vi "Faulhaber_Standalone.vi"() -> ()   [LabVIEW 2011]
panel:
  in  "1:x":i32(slide)=700 scale=-250000.0..250000.0
  in  "Tab Control":enum32{"command", "Script"}(tab)
  in  "commands":cluster{"command":string, "Value":dbl}[](array[cluster])=[{"command"="CONTMOD", "Value"=nan}, {"command"="LR0", "Value"=nan}, {"command"="EN", "Value"=nan}, {"command"="POS", "Value"=nan}, {"command"="OST", "Value"=nan}, {"command"="GAC", "Value"=nan}, {"command"="ac", "Value"=5000.0}, {"command"="GDEC", "Value"=nan}, {"command"="DEC", "Value"=5000.0}, {"command"="GSP", "Value"=nan}, {"command"="SP", "Value"=2500.0}, {"command"="GPOR", "Value"=nan}, {"command"="POR", "Value"=5.0}, {"command"="GI", "Value"=nan}, {"command"="I", "Value"=30.0}, {"command"="GPP", "Value"=nan}, {"command"="PP", "Value"=60.0}, {"command"="GPC", "Value"=nan}, {"command"="LPC", "Value"=500.0}, {"command"="GCC", "Value"=nan}, {"command"="GNL", "Value"=nan}, {"command"="GPL", "Value"=nan}, {"command"="LL", "Value"=12345678.0}, {"command"="TEM", "Value"=nan}, {"command"="GSTN", "Value"=nan}, {"command"="GDP", "Value"=nan}] {"Value" format="%#_8g"}
  in  "Run":bool[](array[boolean])=[FALSE, FALSE, FALSE, FALSE, FALSE, FALSE, FALSE, FALSE, FALSE, FALSE, FALSE, FALSE, FALSE, FALSE, FALSE, FALSE, FALSE, FALSE, FALSE, FALSE, FALSE, FALSE, FALSE]
  out "return name":string="5000\r\n"
  out "return":dbl format="%#_8g"
  out "U16":u16 format="%016x"
  out "Binary":bool[](array[boolean])
  out "Cluster 2":T1={"command"="goto abs", "Numeric"=0.0, "wait ms"=1000, "expected ssi"=235298.717399, "String"="go to low"}
  in  "start":bool
  out "Waveform Chart":dbl(graph)=2342.2826010000135
  in  "Timeout ms":i32=-1
  in  "Export ascii":bool
  in  "read ascii":bool
  in  "Next#":i32=259
  in  "List":T2(array[cluster])=[{"command"="LA", "Numeric"=30000.0, "wait ms"=10, "expected ssi"=0.0, "String"=""}, {"command"="M", "Numeric"=nan, "wait ms"=1000, "expected ssi"=0.0, "String"=""}, {"command"="LA", "Numeric"=0.0, "wait ms"=10, "expected ssi"=0.0, "String"=""}, {"command"="M", "Numeric"=nan, "wait ms"=1000, "expected ssi"=0.0, "String"=""}, {"command"="LA", "Numeric"=-30000.0, "wait ms"=10, "expected ssi"=0.0, "String"=""}, {"command"="M", "Numeric"=nan, "wait ms"=1000, "expected ssi"=0.0, "String"=""}, {"command"="LA", "Numeric"=0.0, "wait ms"=10, "expected ssi"=0.0, "String"=""}, {"command"="M", "Numeric"=nan, "wait ms"=1000, "expected ssi"=0.0, "String"=""}]
  in  "allowed ssi error":dbl=2000.0
  out "ssi in range":bool
  out "connect OK":bool
  out "error out":errorcluster
  in  "stop":bool
  in  "Axis # (-1=aus)":i16=-1
  in  "Port, enter before start":refnum<visa-resource-name>="COM10"
  # "christianb:com10,D:com8"
  # "60000=10mm"
  # "closes comport\notherwise use STOP"
  # "1:x\n2:y\n3:z"
  # "6\n+lim"
  # "7\n-limit"
  # "9\nmotion\ncomplete"
  # "15\nUpdate"
  # "13\nAxisOn"
  # "0\ninit"
  # "Einschalten\nCONTMOD\nLR0  damit keine fahrt\nEN\n\nHO 123"
  # "Parameter\nAC 5000\nDEC 5000\nSP 3000 (RPM=25mm/s)"
  # "software limits: GNL, GPL\nSet LL<0, LL>0\nTEM Temperatur\nLPC 500  (mA)"
  # "Abfragen:\nPOS\nGAC\nGSP\nGRC  aktuelleer Strom\nG..."
  # "Fahren:\nLA 12345\nM"
  # "-1 = stop\n>=0 restart"
  # "NaN expectet will not be checked"
  # "verlorener schritt=256*4 ysteps\nhalber ~200ssi (400 z)"
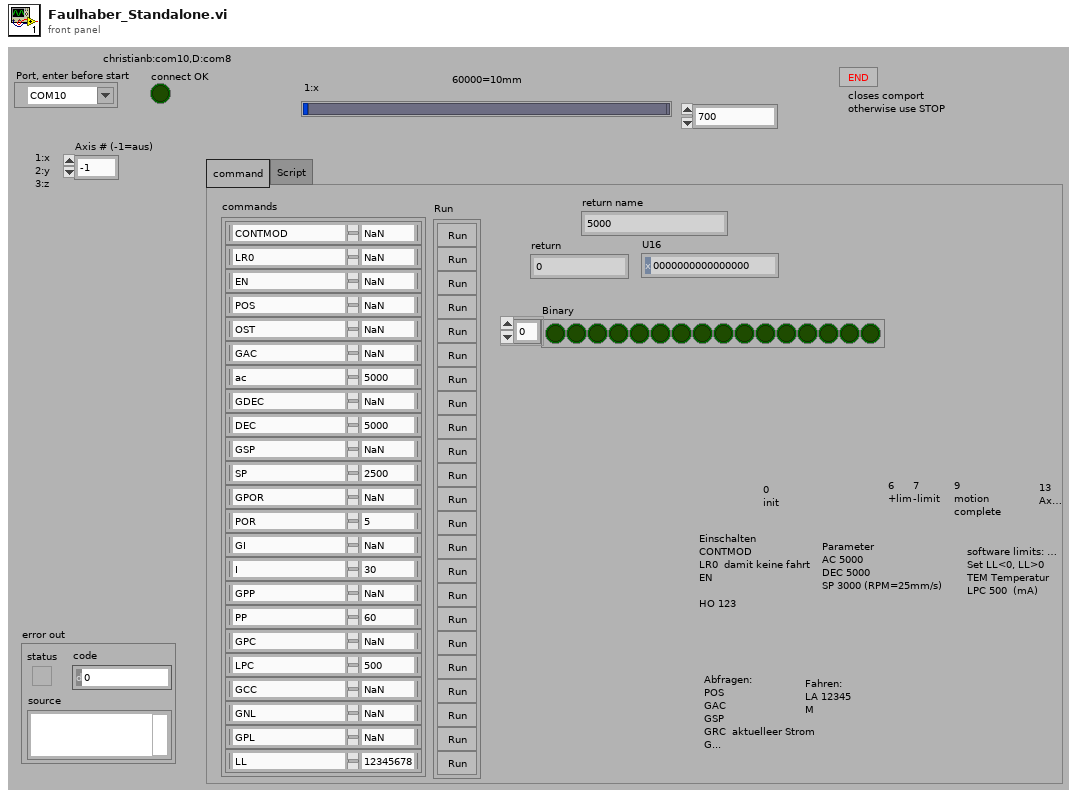
[diagram p1: front panel]
types:
  T1 = cluster{"command":string, "Numeric":dbl, "wait ms":i32, "expected ssi":dbl, "String":string}
  T2 = cluster{"command":string, "Numeric":dbl, "wait ms":i32, "expected ssi":dbl, "String":string}[]
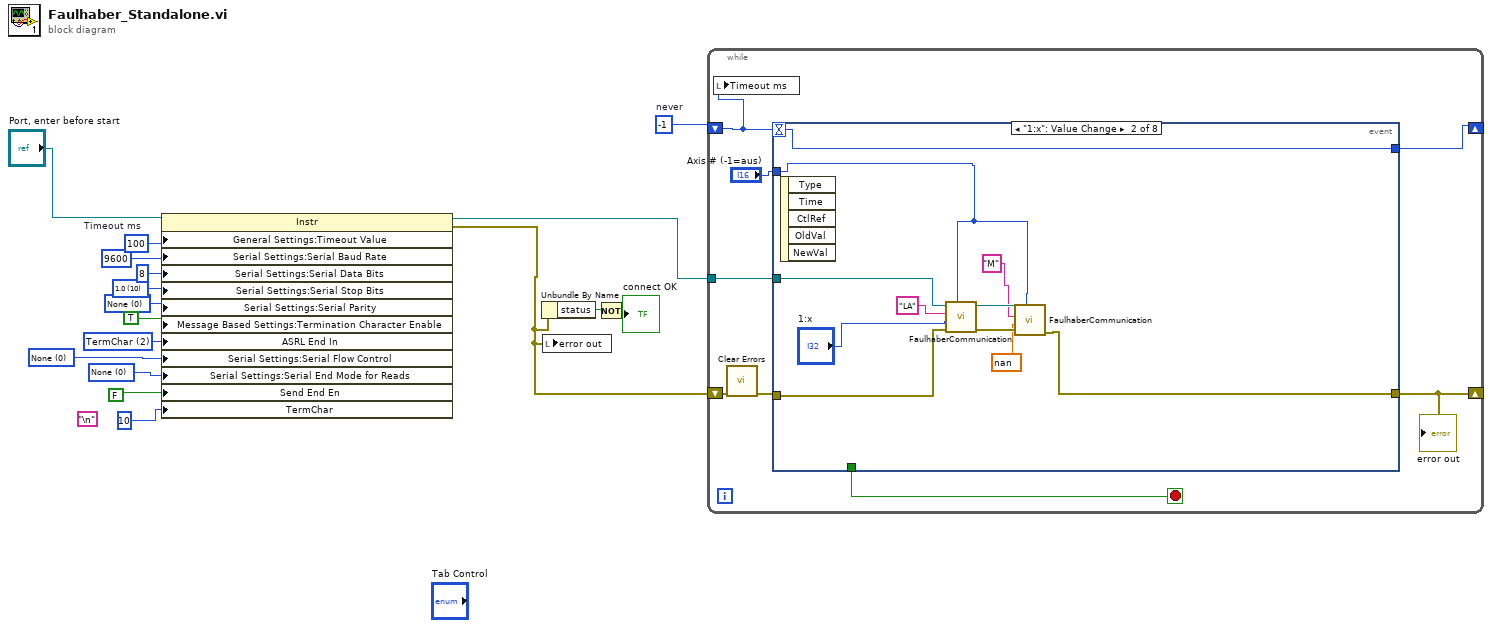
[diagram p0: block diagram]
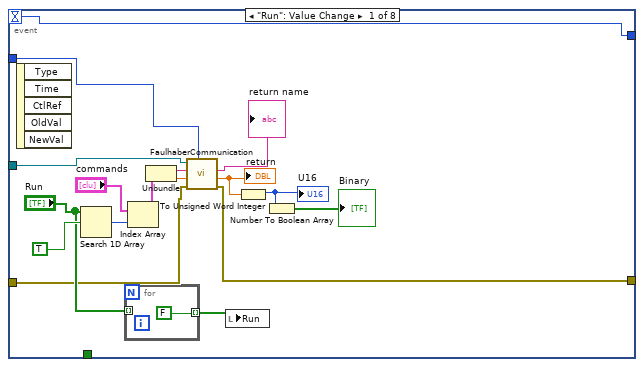
[diagram p2: hidden frame]
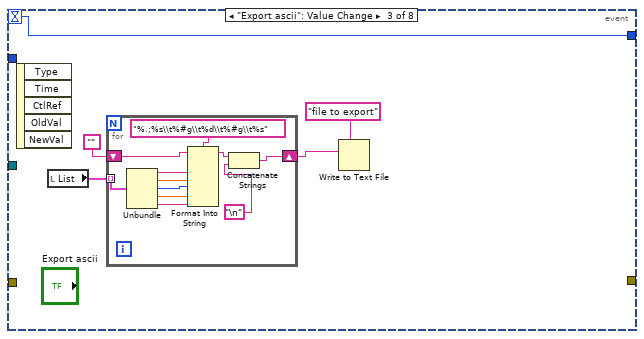
[diagram p3: hidden frame]
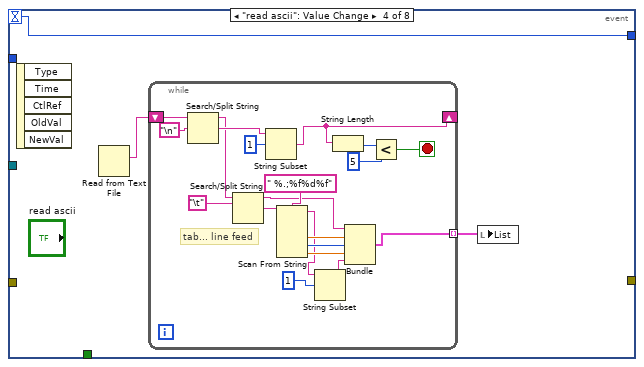
[diagram p4: hidden frame]
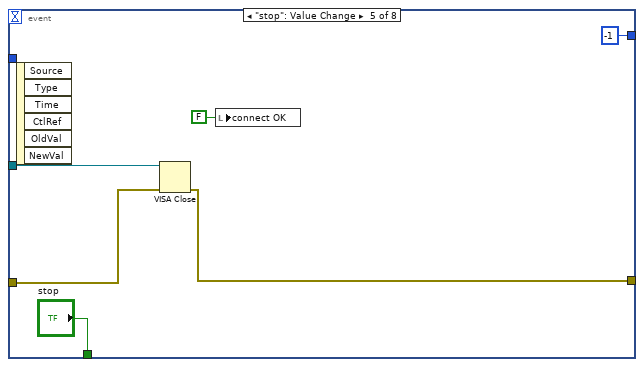
[diagram p5: hidden frame]
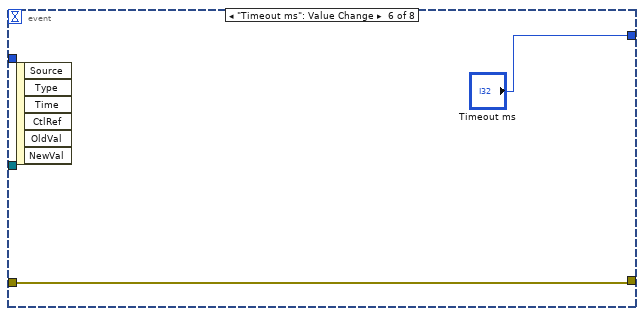
[diagram p6: hidden frame]
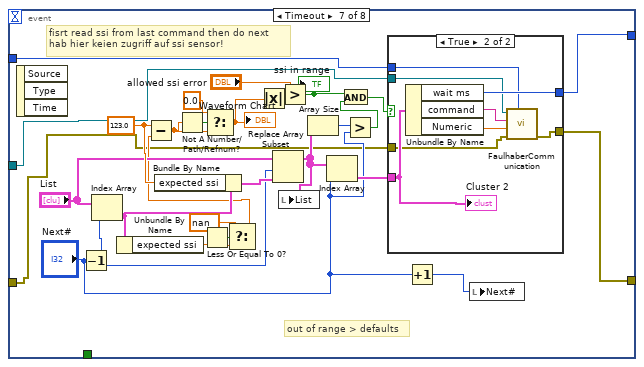
[diagram p7: hidden frame]
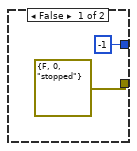
[diagram p8: hidden frame]
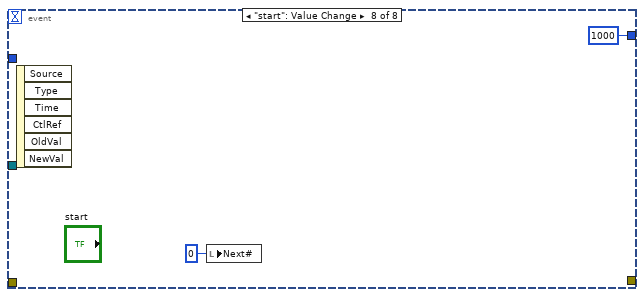
[diagram p9: hidden frame]
diagram:
  (unwired) "\n"
  w3 = u16 2 items=["None", "Last Bit", "TermChar"] ("Serial Settings:End Mode for Reads")
  w9 = u32 100  # Timeout ms
  w11 = u16 10 items=["1.0"=10, "1.5"=15, "2.0"=20] ("Serial Settings:Stop Bits")
  w12 = u16 0 items=["None", "Odd", "Even", "Mark", "Space"] ("Serial Settings:Parity")
  w13 = u16 0 items=["None", "Last Bit", "TermChar"] ("Serial Settings:End Mode for Reads")
  w4 = u16 0 items=["None", "XON/XOFF", "RTS/CTS", "XON/XOFF & RTS/CTS", "DTR/DSR", "XON/XOFF & DTR/DSR"] ("Serial Settings:Flow Control")
  w15 = -1  # never
  n1 = property class="Instr"(reference="Port, enter before start", "General Settings:Timeout Value"=w9, "Serial Settings:Serial Baud Rate"=u32 9600 ("Serial Settings:Baud Rate"), "Serial Settings:Serial Data Bits"=u16 8 ("Serial Settings:Data Bits"), "Serial Settings:Serial Stop Bits"=w11, "Serial Settings:Serial Parity"=w12, "Message Based Settings:Termination Character Enable"=TRUE, "ASRL End In"=w3, "Serial Settings:Serial Flow Control"=w4, "Serial Settings:Serial End Mode for Reads"=w13, "Send End En"=FALSE ("Message Based Settings:Send End Enable"), "TermChar"=u8 10 ("Message Based Settings:Termination Character")) -> (reference out=w5:refnum<visa-resource-name>, error out=w1:errorcluster)  [unwired: 1 in]
  n2 = Unbundle By Name(w1) -> ("status"=w17:bool)
  n3 = local write "error out"(w1) -> ()
  n4 = Not(x=w17) -> (.not. x?=→"connect OK":bool)
  n5 = while {
    shift-right: [w24] -> _
    shift-left: w1 -> [w23]
    tunnel: w5 -> [w22]
    shift-right: [w18] -> _
    shift-left: w15 -> [w19]
    stop <- w25 stop-if-true
    n6 = local write "Timeout ms"(w19) -> ()
    n7 = call <vilib>:"Clear Errors.vi"("error in (no error)"=w23) -> ("error out"=w21:errorcluster)  [unwired: 6 out]
    n8 = event shown="[1] \"1:x\": Value Change" {
      selector: _ -> [_ _ _ _ _ _ _ _]
      dyn-events: _ -> [_ _ _ _ _ _ _ _]
      timeout: w19 -> [w34 w54 w55 w71 _ _ _ _]
      tunnel: [_ _ _ _ "stop" _ _ _] -> w25
      tunnel: [w28 w47 _ _ w97 w100 w119 _] -> w24
      tunnel: w21 -> [w33 w52 _ _ w98 w100 w102 _]
      tunnel: w22 -> [w32 w53 _ _ w96 _ w103 _]
      tunnel: "Axis # (-1=aus)" -> [w29 w44 _ _ _ _ w122 _]
      tunnel: [w34 w54 w55 w71 -1 ("wait ms") "Timeout ms" w120 1000 ("wait ms")] -> w18
      event "Run": Value Change {
        n9 = event-data() -> ()  [unwired: 6 out]
        n10 = Search 1D Array(1D array="Run", element=TRUE) -> (index of element=w39:i32)  [unwired: 1 out]
        n11 = for {
          tunnel: "Run" -> [_] mode=indexing
          tunnel: [FALSE ("element")] -> w35 mode=indexing
        }
        n12 = Index Array(array="commands", index=w39) -> (element=w37:cluster{"command":string, "Value":dbl})
        n13 = Unbundle(w37) -> ("command"=w31:string, "Value"=w30:dbl)
        n14 = call "FaulhaberCommunication.vi"("axis-optional-1"=w29, "error in (no error)"=w33, "Argument-optional"=w30, "Befehl"=w31, "VISA resource name"=w32) -> ("error out"=w28:errorcluster, 1:"return"=w27:dbl, 2:"return"=→"return name":string)  [unwired: 3 in, 1 out]
        "return" <- w27
        n15 = local write "Run"(w35) -> ()
        n16 = To Unsigned Word Integer(number=w27) -> (unsigned 16bit integer=w42:u16)
        "U16" <- w42
        n17 = Number To Boolean Array(number=w42) -> (Boolean array=→"Binary":bool[])
      }
      event "1:x": Value Change {
        n18 = event-data() -> ()  [unwired: 6 out]
        n19 = call "FaulhaberCommunication.vi"("axis-optional-1"=w44, "error in (no error)"=w52, "Argument-optional"="1:x", "Befehl"="LA" ("command"), "VISA resource name"=w53) -> ("error out"=w48:errorcluster, "VISA resource name out"=w49:refnum<visa-resource-name>)  [unwired: 3 in, 2 out]
        n20 = call "FaulhaberCommunication.vi"("axis-optional-1"=w44, "error in (no error)"=w48, "Argument-optional"=nan ("Argument-optinal"), "Befehl"="M" ("command"), "VISA resource name"=w49) -> ("error out"=w47:errorcluster)  [unwired: 3 in, 3 out]
      }
      event "Export ascii": Value Change {
        n21 = event-data() -> ()  [unwired: 6 out]
        n22 = local read "List"() -> (w59:T2)
        n23 = for {
          tunnel: w59 -> [w70] mode=indexing
          shift-right: [w62] -> w57
          shift-left: "" -> [w69]
          n24 = Unbundle(w70) -> ("command"=w68:string, "Numeric"=w67:dbl, "wait ms"=w66:i32, "expected ssi"=w65:dbl, "String"=w64:string)
          n25 = Format Into String(format string="%.;%s\\t%#g\\t%d\\t%#g\\t%s", initial string=w69, w68, w67, w66, w65, w64) -> (resulting string=w63:string)  [unwired: 1 in, 1 out]
          n26 = Concatenate Strings(w63, "\n") -> (w62:string)
        }
        n27 = Write to Text File(prompt (Choose or enter file path)="file to export", text=w57) -> ()  [unwired: 2 in, 3 out]
      }
      event "read ascii": Value Change {
        n28 = event-data() -> ()  [unwired: 6 out]
        n29 = Read from Text File() -> (text=w73:string)  [unwired: 4 in, 3 out]
        n30 = while {
          shift-right: [w80] -> _
          shift-left: w73 -> [w93]
          tunnel: [w88] -> w72 mode=indexing
          stop <- w77 stop-if-true
          # "tab... line feed"
          n31 = Search/Split String(string=w93, search string/char (-)="\n") -> (substring before match=w82:string, match + rest of string=w86:string)  [unwired: 1 in, 1 out]
          n32 = Search/Split String(string=w82, search string/char (-)="\t") -> (substring before match=w83:string, match + rest of string=w81:string)  [unwired: 1 in, 1 out]
          n33 = String Subset(string=w86, offset (0)=1) -> (substring=w80:string)  [unwired: 1 in]
          n34 = Scan From String(format string=" %.;%f%d%f", input string=w81) -> (remaining string=w75:string, output 1=w91:dbl, output 2=w90:i32, output 3=w89:dbl)  [unwired: 5 in, 2 out]
          n35 = String Subset(string=w75, offset (0)=1) -> (substring=w74:string)  [unwired: 1 in]
          n36 = String Length(string=w80) -> (length=w79:i32)
          n37 = Bundle(w83, w91, w90, w89, w74) -> (w88:cluster{string, dbl, i32, dbl, string})  [unwired: 1 in]
          n38 = Less?(x=w79, y=5) -> (x < y?=w77:bool)
        }
        n39 = local write "List"(w72) -> ()
      }
      event "stop": Value Change {
        n40 = event-data() -> ()  [unwired: 7 out]
        n41 = VISA Close(VISA resource name=w96, error in (no error)=w98) -> (error out=w97:errorcluster)
        n42 = local write "connect OK"(FALSE ("connect OK")) -> ()
      }
      event "Timeout ms": Value Change {
        n43 = event-data() -> ()  [unwired: 7 out]
      }
      event Timeout {
        w126 = 123.0 ("x")
        # "out of range > defaults"
        # "fisrt read ssi from last command then do next\nhab hier keien zugriff auf ssi sensor!"
        n44 = event-data() -> ()  [unwired: 4 out]
        n45 = Decrement(x="Next#") -> (x-1=w123:i32)
        n46 = Index Array(array="List", index=w123) -> (element=w127:T1)
        n47 = Unbundle By Name(w127) -> ("expected ssi"=w108:dbl)
        n48 = Bundle By Name(cluster=w127, "expected ssi"=w126) -> (w124:T1)
        n49 = Less Or Equal To 0?(x=w108) -> (x <= 0?=w109:bool)
        n50 = Select(t=nan, s=w109, f=w108) -> (s? t:f=w107:dbl)
        n51 = Subtract(x=w126, y=w107) -> (x-y=w111:dbl)
        n52 = Not A Number/Path/Refnum?(number/path/refnum=w111) -> (NaN/Path/Refnum?=w112:bool)
        n53 = Select(t=0.0, s=w112, f=w111) -> (s? t:f=w110:dbl)
        "Waveform Chart" <- w110
        n54 = Absolute Value(x=w110) -> (abs(x)=w129:dbl)
        n55 = Replace Array Subset(array="List", new element=w124, index=w123) -> (w118:T2)
        n56 = local write "List"(w118) -> ()
        n57 = Greater?(x="allowed ssi error", y=w129) -> (0:w115:bool)
        "ssi in range" <- w115
        n58 = Array Size(array=w118) -> (size(s)=w117:i32)
        n59 = Index Array(array=w118, index="Next#") -> (element=w121:T1)
        n60 = Greater?(x=w117, y="Next#") -> (0:w116:bool)
        n61 = And(x=w115, y=w116) -> (x .and. y?=w114:bool)
        n62 = case shown="True" w114 {
          tunnel: w122 -> [_ w132]
          tunnel: w103 -> [_ w135]
          tunnel: w121 -> [_ w138]
          tunnel: w102 -> [_ w136]
          tunnel: [-1 ("wait ms") w139] -> w120
          tunnel: [errorcluster {"status"=FALSE, "code"=0, "source"="stopped"} ("error out") w137] -> w119
          frame False {
          }
          frame True {
            n63 = Unbundle By Name(w138) -> ("wait ms"=w139:i32, "command"=w134:string, "Numeric"=w133:dbl)
            n64 = call "FaulhaberCommunication.vi"("axis-optional-1"=w132, "error in (no error)"=w136, "Argument-optional"=w133, "Befehl"=w134, "VISA resource name"=w135) -> ("error out"=w137:errorcluster)  [unwired: 3 in, 3 out]
            "Cluster 2" <- w138
          }
        }
        n65 = Increment(x="Next#") -> (x+1=w104:i32)
        n66 = local write "Next#"(w104) -> ()
      }
      event "start": Value Change {
        n67 = event-data() -> ()  [unwired: 7 out]
        n68 = local write "Next#"(0 ("Next#")) -> ()
      }
    }
    "error out" <- w24
  }
